vi "Sense.ParseStream.vi"(1 "UART Stream":u8[](array[numeric])) -> (0 "Streaming Data":T1)   [LabVIEW 2010]
uses:
  Streaming Data.ctl
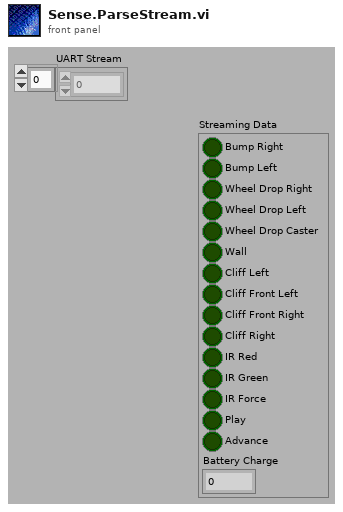
[diagram p1: front panel]
types:
  T1 = typedef "Streaming Data.ctl" = cluster{"Bump Right":bool, "Bump Left":bool, "Wheel Drop Right":bool, "Wheel Drop Left":bool, "Wheel Drop Caster":bool, "Wall":bool, "Cliff Left":bool, "Cliff Front Left":bool, "Cliff Front Right":bool, "Cliff Right":bool, "IR Red":bool, "IR Green":bool, "IR Force":bool, "Play":bool, "Advance":bool, "Battery Charge":i16}
  T2 = typedef "iRobot Bumps + Wheel Drops.ctl" = cluster{"Wheeldrop Caster":bool, "Wheeldrop Left":bool, "Wheeldrop Right":bool, "Bump Left":bool, "Bump Right":bool}
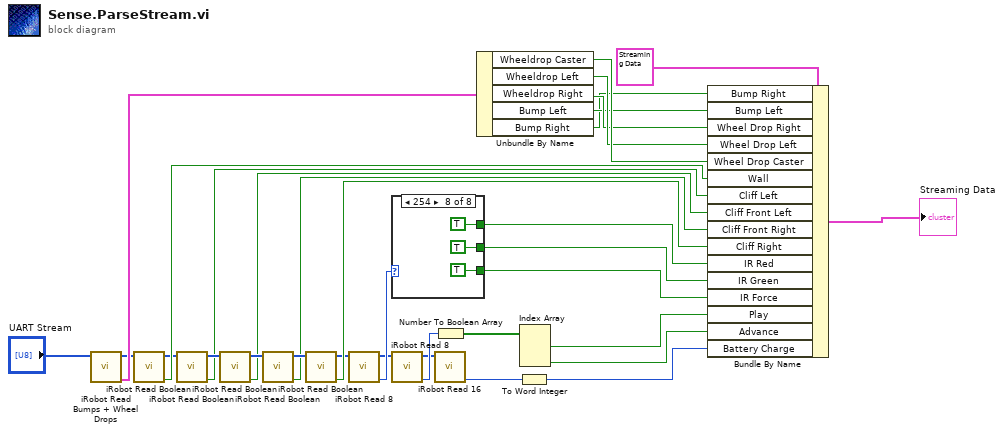
[diagram p0: block diagram]
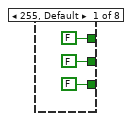
[diagram p2: hidden frame]
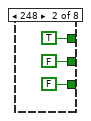
[diagram p3: hidden frame]
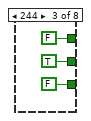
[diagram p4: hidden frame]
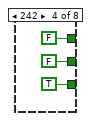
[diagram p5: hidden frame]
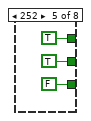
[diagram p6: hidden frame]
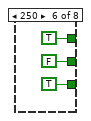
[diagram p7: hidden frame]
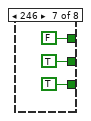
[diagram p8: hidden frame]
diagram:
  n1 = call "iRobot Read Bumps + Wheel Drops.vi"("stream in"="UART Stream") -> ("Bumps + Wheel Drops"=w6:T2, "stream out"=w2:u8[])  [unwired: 9 out]
  n2 = call "iRobot Read Boolean.vi"("stream in"=w2) -> ("Value"=w12:bool, "stream out"=w5:u8[])  [unwired: 9 out]
  n3 = call "iRobot Read Boolean.vi"("stream in"=w5) -> ("Value"=w13:bool, "stream out"=w14:u8[])  [unwired: 9 out]
  n4 = call "iRobot Read Boolean.vi"("stream in"=w14) -> ("Value"=w15:bool, "stream out"=w16:u8[])  [unwired: 9 out]
  n5 = call "iRobot Read Boolean.vi"("stream in"=w16) -> ("Value"=w17:bool, "stream out"=w21:u8[])  [unwired: 9 out]
  n6 = call "iRobot Read Boolean.vi"("stream in"=w21) -> ("Value"=w23:bool, "stream out"=w22:u8[])  [unwired: 9 out]
  n7 = call "iRobot Read 8.vi"("stream in"=w22) -> ("value"=w20:u8, "stream out"=w18:u8[])  [unwired: 9 out]
  n8 = case shown="254" w20 {
    tunnel: [FALSE TRUE FALSE FALSE TRUE TRUE FALSE TRUE] -> w24
    tunnel: [FALSE FALSE TRUE FALSE TRUE FALSE TRUE TRUE] -> w25
    tunnel: [FALSE FALSE FALSE TRUE FALSE TRUE TRUE TRUE] -> w26
    frame 255, Default {
    }
    frame 248 {
    }
    frame 244 {
    }
    frame 242 {
    }
    frame 252 {
    }
    frame 250 {
    }
    frame 246 {
    }
    frame 254 {
    }
  }
  n9 = call "iRobot Read 8.vi"("stream in"=w18) -> ("value"=w27:u8, "stream out"=w19:u8[])  [unwired: 9 out]
  n10 = call "iRobot Read 16.vi"("stream in"=w19) -> ("value"=w31:u16)  [unwired: 10 out]
  n11 = Number To Boolean Array(number=w27) -> (Boolean array=w28:bool[])
  n12 = Unbundle By Name(w6) -> ("Wheeldrop Caster"=w11:bool, "Wheeldrop Left"=w10:bool, "Wheeldrop Right"=w9:bool, "Bump Left"=w8:bool, "Bump Right"=w7:bool)
  n13 = To Word Integer(number=w31) -> (16bit integer=w32:i16)
  n14 = Index Array(array=w28) -> (element #1=w29:bool, element #3=w30:bool)  [unwired: 3 in, 1 out]
  n15 = Bundle By Name(cluster=T1 {"Bump Right"=FALSE, "Bump Left"=FALSE, "Wheel Drop Right"=FALSE, "Wheel Drop Left"=FALSE, "Wheel Drop Caster"=FALSE, "Wall"=FALSE, "Cliff Left"=FALSE, "Cliff Front Left"=FALSE, "Cliff Front Right"=FALSE, "Cliff Right"=FALSE, "IR Red"=FALSE, "IR Green"=FALSE, "IR Force"=FALSE, "Play"=FALSE, "Advance"=FALSE, "Battery Charge"=0} ("Streaming Data"), "Bump Right"=w7, "Bump Left"=w8, "Wheel Drop Right"=w9, "Wheel Drop Left"=w10, "Wheel Drop Caster"=w11, "Wall"=w12, "Cliff Left"=w13, "Cliff Front Left"=w15, "Cliff Front Right"=w17, "Cliff Right"=w23, "IR Red"=w24, "IR Green"=w25, "IR Force"=w26, "Play"=w29, "Advance"=w30, "Battery Charge"=w32) -> (→"Streaming Data":T1)
